vi "Manipulator.vi"(10 "Manipulator On":bool, 11 "Ball Queued":bool) -> (1 "Ball Queue Voltage":dbl, 2 "Inside Manupulator Voltage":dbl, 3 "Outisde Manipulator Voltage":dbl)   [LabVIEW 2016]
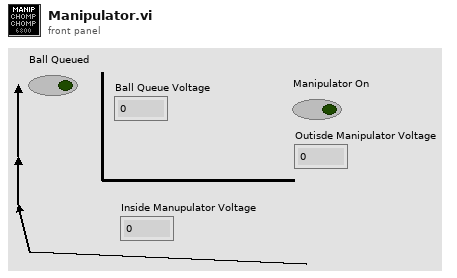
[diagram p1: front panel]
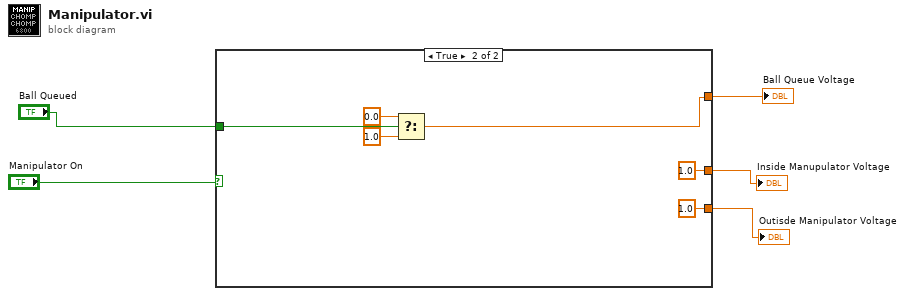
[diagram p0: block diagram]
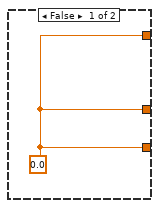
[diagram p2: hidden frame]
diagram:
  n1 = case shown="True" "Manipulator On" {
    tunnel: [w6 w7] -> w4
    tunnel: [w6 1.0 ("Ball Queue Voltage")] -> w3
    tunnel: [w6 1.0 ("Ball Queue Voltage")] -> w2
    tunnel: "Ball Queued" -> [_ w10]
    frame False {
      w6 = 0.0 ("Ball Queue Voltage")
    }
    frame True {
      n2 = Select(t=0.0, s=w10, f=1.0) -> (s? t:f=w7:dbl)
    }
  }
  "Outisde Manipulator Voltage" <- w2
  "Inside Manupulator Voltage" <- w3
  "Ball Queue Voltage" <- w4
